vi "Test App Set Duplicate Process.vi"(8 "error in (no error)":errorcluster, 11 "Rig Test in":refnum<class "Application Test.lvclass">) -> (0 "error out":errorcluster, 3 "Rig Test out":refnum<class "Application Test.lvclass">)   [LabVIEW 2020, in "Application Test.lvclass"]
uses:
  Application Test.lvclass
  C:/Program Files (x86)/National Instruments/LabVIEW 2020/vi.lib/Asteme/LUnit/Test Case.lvclass
  Framework/Process/Process.lvclass
  Framework/Process/Process.lvclass/Process.ctl
  Framework/Application/Application.lvclass/Application.ctl
  <vilib>/Asteme/LUnit/Test Case.lvclass/Test Case.ctl
  <vilib>/Asteme/LUnit/LUnit Assertion Result.lvclass/LUnit Assertion Result.ctl
  Framework/Application/Private/Add Process to Map.vi
  Framework/Process/Protected/Messaging/Enqueue Message.vi
  Framework/Process/Protected/SubVIs/Set Context.vi
  Framework/Process/Public/Lifecycle/Get Lifecycle State.vi
  Framework/Process/Protected/Messaging/Request Message.vi
  <vilib>/Asteme/LUnit/Palette/Pass.vi
  <vilib>/Asteme/LUnit/Palette/Fail.vi
  <vilib>/Asteme/LUnit/Variant to string.vi
  <vilib>/Asteme/LUnit/Set Assertion Type.vi
  Framework/Process/Private/SubVIs/Wait for finish.vi
  Framework/Process/Private/SubVIs/Set Lifecycle State.vi
  <vilib>/Utility/error.llb/Clear Errors.vi
  Framework/Process/Community/Leave Process Loop.vi
  Framework/Process/Private/SubVIs/Enqueue Request Message.vi
  <vilib>/Asteme/LUnit/Add test result.vi
  <vilib>/Asteme/LUnit/LUnit Write Passed.vi
  <vilib>/Asteme/LUnit/LUnit Get Test Case.vi
  <vilib>/Asteme/LUnit/Assertion Result/LUnit Get Test Name.vi
  <vilib>/Asteme/LUnit/LUnit Write Message.vi
  <vilib>/Asteme/LUnit/LUnit Write Description.vi
  <vilib>/Asteme/LUnit/LUnit Write Assertion Type.vi
  <vilib>/Asteme/LUnit/Read Test Case Name.vi
  Framework/Application/Application.lvclass
  C:/Users/anton/Documents/GitHub/Triarc-Framework/source/Framework/Process/Process.lvclass
  <vilib>/Utility/error.llb/Error Cluster From Error Code.vi
  Framework/Application/Private/Update Context for Owned Processes.vi
  Framework/Process/Private/SubVIs/Wait for Response Message.vi
  <vilib>/Utility/Data Type/Get Type Information.vi
  <vilib>/Utility/LVClass/Get LV Class Name.vi
  <vilib>/Asteme/LUnit/LUnit Assertion Result.lvclass
  <vilib>/Asteme/LUnit/Test Case.lvclass
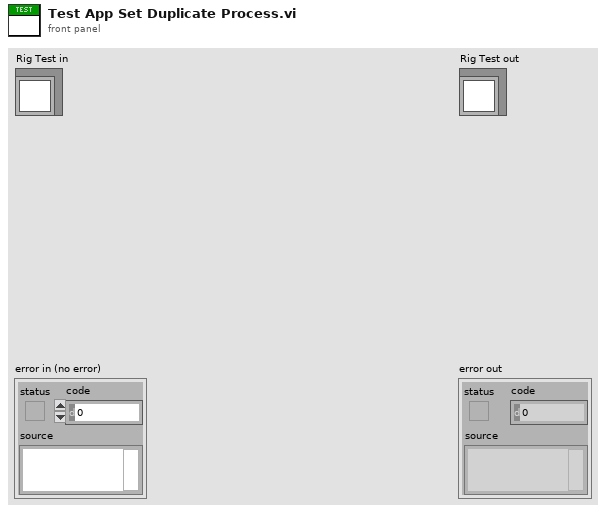
[diagram p1: front panel]
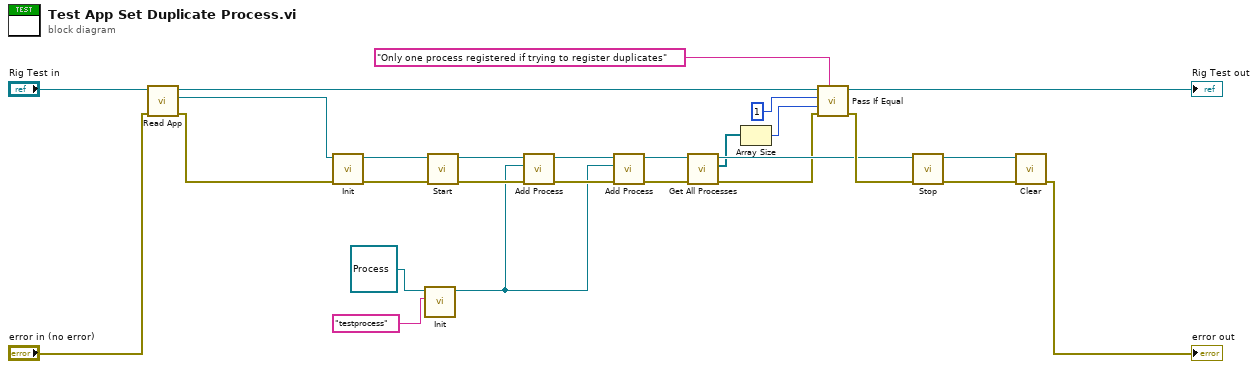
[diagram p0: block diagram]
diagram:
  n1 = call "Read App.vi"("error in (no error)"="error in (no error)", "Application Test In"="Rig Test in") -> ("error out"=w2:errorcluster, "App out"=w1:refnum<class "Application.lvclass">, "Application Test Out"=w19:refnum<class "Application Test.lvclass">)  [unwired: 7 in]
  n2 = call-dynamic "Init.vi"("error in (no error)"=w2, "Process In"=w1) -> ("error out"=w14:errorcluster, "Process Out"=w24:refnum<class "Application.lvclass">)  [unwired: 8 in]
  n3 = call-dynamic "Init.vi"("Name"="testprocess", "Process In"=refnum<class "Process.lvclass"> refnum ("Process.lvclass")) -> ("Process Out"=w12:refnum<class "Process.lvclass">)  [unwired: 8 in, 1 out]
  n4 = call "Start.vi"("error in (no error)"=w14, "Process In"=w24) -> ("error out"=w13:errorcluster, "Process Out"=w15:refnum<class "Application.lvclass">)  [unwired: 8 in]
  n5 = call "Add Process.vi"("error in (no error)"=w13, "Process"=w12, "Rig In"=w15) -> ("error out"=w20:errorcluster, "Rig Out"=w23:refnum<class "Application.lvclass">)  [unwired: 7 in]
  n6 = call "Add Process.vi"("error in (no error)"=w20, "Process"=w12, "Rig In"=w23) -> ("error out"=w10:errorcluster, "Rig Out"=w25:refnum<class "Application.lvclass">)  [unwired: 7 in]
  n7 = call "Get All Processes.vi"("error in (no error)"=w10, "Application In"=w25) -> ("error out"=w9:errorcluster, "App Processes"=w8:refnum<class "Process.lvclass">[], "Application Out"=w11:refnum<class "Application.lvclass">)  [unwired: 7 in]
  n8 = Array Size(array=w8) -> (size(s)=w7:i32)
  n9 = call <vilib>:"Pass If Equal.vi"("Description"="Only one process registered if trying to register duplicates", "error in (no error)"=w9, "Actual"=w7, "Expected"=1 ("size(s)"), "Test Case In"=w19) -> ("error out"=w17:errorcluster, "Test Case Out"=→"Rig Test out":refnum<class "Application Test.lvclass">)  [unwired: 5 in]
  n10 = call "Stop.vi"("error in (no error)"=w17, "Process In"=w11) -> ("error out"=w4:errorcluster, "Process Out"=w5:refnum<class "Application.lvclass">)  [unwired: 7 in, 1 out]
  n11 = call-dynamic "Clear.vi"("error in (no error)"=w4, "Application In"=w5) -> ("error out"=→"error out":errorcluster)  [unwired: 8 in, 1 out]
